vi "sub_automatic_voltage_set.vi"(8 "Suppressor new [V]":dbl, 9 "Suppressor old [V]":dbl, 10 "Tip new [V]":dbl, 11 "Tip old [V]":dbl) -> (0 "error out":errorcluster)   [LabVIEW 2009]
panel:
  in  "max Spanungsdifferenz":dbl
  in  "Schritte pro Sec":dbl
  in  "Geschw. [V/s]":dbl
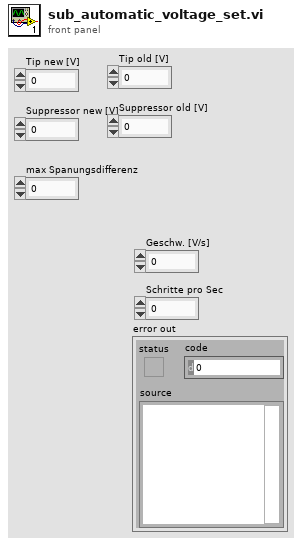
[diagram p1: front panel]
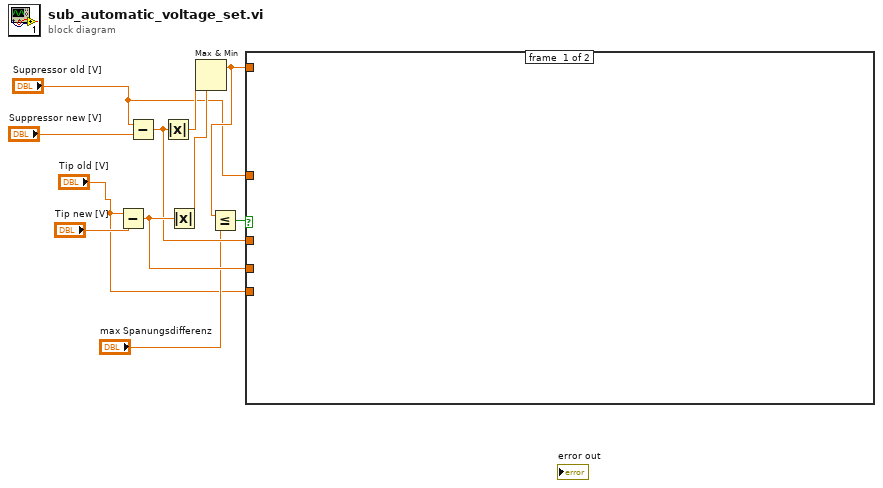
[diagram p0: block diagram]
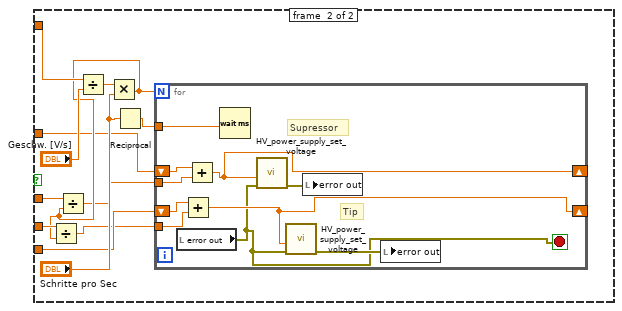
[diagram p2: hidden frame]
diagram:
  n1 = Subtract(x="Tip old [V]", y="Tip new [V]") -> (x-y=w9:dbl)
  n2 = Subtract(x="Suppressor old [V]", y="Suppressor new [V]") -> (x-y=w8:dbl)
  n3 = Absolute Value(x=w8) -> (abs(x)=w6:dbl)
  n4 = Absolute Value(x=w9) -> (abs(x)=w7:dbl)
  n5 = Max & Min(x=w6, y=w7) -> (max(x,y)=w4:dbl)  [unwired: 1 out]
  n6 = Less Or Equal?(x=w4, y="max Spanungsdifferenz") -> (x <= y?=w5:bool)
  n7 = case shown="True" w5 {
    tunnel: w9 -> [_ w17]
    tunnel: w8 -> [_ w18]
    tunnel: w4 -> [_ w19]
    tunnel: "Suppressor old [V]" -> [_ w15]
    tunnel: "Tip old [V]" -> [_ w14]
    frame #0 {
    }
    frame #1 {
      n8 = Divide(x=w19, y="Geschw. [V/s]") -> (x/y=w23:dbl)
      n9 = Multiply(x=w23, y="Schritte pro Sec") -> (x*y=w16:dbl)
      n10 = Divide(x=w17, y=w16) -> (x/y=w12:dbl)
      n11 = Divide(x=w18, y=w16) -> (x/y=w13:dbl)
      n12 = Reciprocal(x="Schritte pro Sec") -> (1/x=w20:dbl)
      n13 = for {
        N: w16 -> [_]
        tunnel: w20 -> [w33]
        shift-right: [w28] -> _
        shift-left: w15 -> [w30]
        shift-right: [w25] -> _
        shift-left: w14 -> [w27]
        tunnel: w13 -> [w29]
        tunnel: w12 -> [w26]
        stop <- w24 stop-if-true
        # "Tip"
        # "Supressor"
        n14 = local read "error out"() -> (w24:errorcluster)
        n15 = Add(x=w27, y=w26) -> (x+y=w25:dbl)
        n16 = Add(x=w30, y=w29) -> (x+y=w28:dbl)
        n17 = Wait (ms)(milliseconds to wait=w33) -> ()  [unwired: 1 out]
        n18 = call "HV_power_supply_set_voltage.vi"("error in"=w24, "Desired output voltage in V (HV power supply)"=w28) -> ("error out"=w31:errorcluster)  [unwired: 8 in]
        n19 = call "HV_power_supply_set_voltage.vi"("error in"=w24, "Desired output voltage in V (HV power supply)"=w25) -> ("error out"=w32:errorcluster)  [unwired: 8 in]
        n20 = local write "error out"(w31) -> ()
        n21 = local write "error out"(w32) -> ()
      }
    }
  }
